vi "subGenerateDGMLOtherFilesFolderString.vi"(7 "ILabVIEWItem in":refnum<class "ILabVIEWItem.lvclass">, 8 "Links in":T1, 9 "Nodes in":T1, 11 "CGrapherDGML in":refnum<class "CGrapherDGML.lvclass">) -> (0 "Links":T1, 1 "Nodes":T1, 2 "Path":string="Z:\\OtherFiles", 3 "CGrapherDGML":refnum<class "CGrapherDGML.lvclass">)   [LabVIEW 2020, in "DefaultExtensions.lvlib" / "CGrapherDGML.lvclass"]
uses:
  CGrapherDGML.lvclass
  obj/Addons/LabVIEWObjectInterfaces.lvlibp/LabVIEWObjectInterfaces/ILabVIEWItem/ILabVIEWItem.lvclass
  obj/Addons/LabVIEWItem.lvlibp/LabVIEWItem/CLabVIEWItem/ConnectionSet.ctl
  ecf4d353-cf80-4459-a486-8bebc84a9ab0.vi
  obj/Addons/LabVIEWItem.lvlibp/LabVIEWItem/CLabVIEWItem/CLabVIEWItem.lvclass
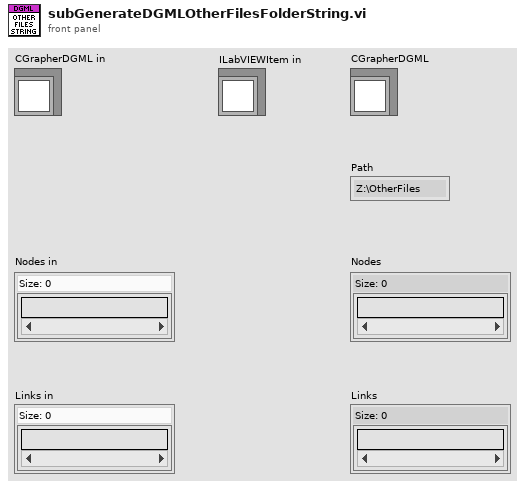
[diagram p1: front panel]
types:
  T1 = typedef "LabVIEWItem.lvlibp/CLabVIEWItem.lvclass/ConnectionSet.ctl" = set{string}
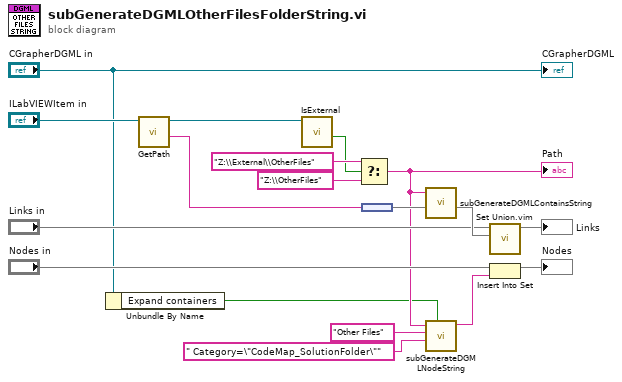
[diagram p0: block diagram]
diagram:
  n1 = Unbundle By Name("CGrapherDGML in") -> ("Expand containers"=w1:bool)
  n2 = call-dynamic "GetPath.vi"("ILabVIEWItem in"="ILabVIEWItem in") -> ("Path"=w18:string, "ILabVIEWItem out"=w12:refnum<class "ILabVIEWItem.lvclass">)  [unwired: 8 in, 1 out]
  n3 = call-dynamic "IsExternal.vi"("ILabVIEWItem in"=w12) -> ("Is external?"=w4:bool)  [unwired: 8 in, 2 out]
  n4 = Select(t="Z:\\External\\OtherFiles" ("format string"), s=w4, f="Z:\\OtherFiles" ("format string")) -> (s? t:f=w3:string)
  "Path" <- w3
  n5 = node(w18) -> (w17:set{string})
  n6 = call "subGenerateDGMLContainsString.vi"("Contained"=w17, "Source"=w3) -> ("Links"=w16:T1)  [unwired: 9 in]
  n7 = call "subGenerateDGMLNodeString.vi"("Expand?"=w1, "Code schema"=" Category=\"CodeMap_SolutionFolder\"" ("format string"), "Label"="Other Files" ("format string"), "Id"=w3) -> ("Node string"=w14:string)  [unwired: 7 in]
  n8 = call "Set Union.vim"("set 2"=w16, "set 1"="Links in") -> ("union"=→"Links":T1)  [unwired: 9 in]
  n9 = Insert Into Set(10:w14, 11:"Nodes in") -> (3:→"Nodes":T1)  [unwired: 1 out]
  "CGrapherDGML" <- "CGrapherDGML in"
